vi "ROI entry-Check Z range and adjust.vi"(10 "ROI File data":dbl[][](array[numeric]), 11 "Old ROI file path":path) -> (2 "Adjusted ROI Data":dbl[][](array[numeric]), 3 "Latest AOL Z values":dbl[](array[numeric]))   [LabVIEW 2017]
uses:
  Typedefs/fgv_actions.ctl
panel:
  out "error out":errorcluster
  in  "error in (no error)":errorcluster
  in  "Loaded ROI Z Stop Values":dbl[](array[numeric])
  out "ROI Z stop (coerced)":dbl[](array[numeric])
  out "Z Stop Array":dbl[](array[numeric])
  out "Z Stop Code":u8[](array[numeric])
  out "Z start code":u8[](array[numeric])
  out "Z Start Array":dbl[](array[numeric])
  out "ROI Z start (coerced)":dbl[](array[numeric])
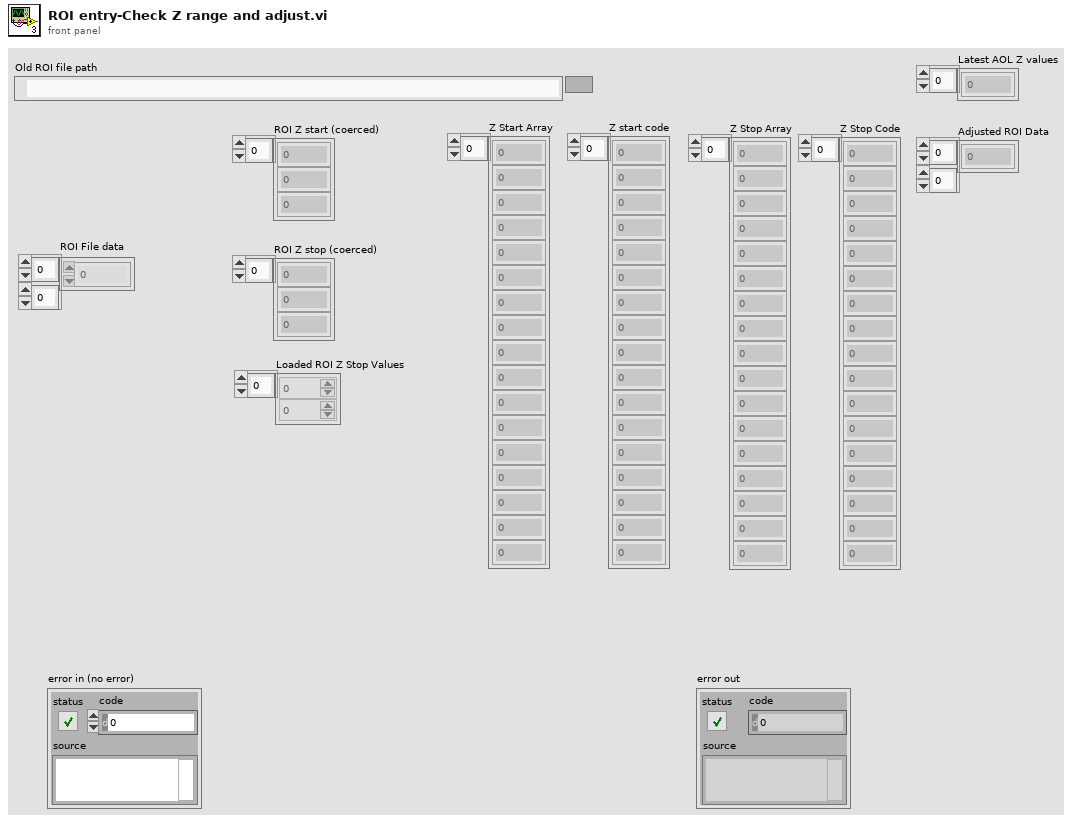
[diagram p1: front panel]
types:
  T1 = typedef "fgv_actions.ctl" = enum16{"Get", "Set"}
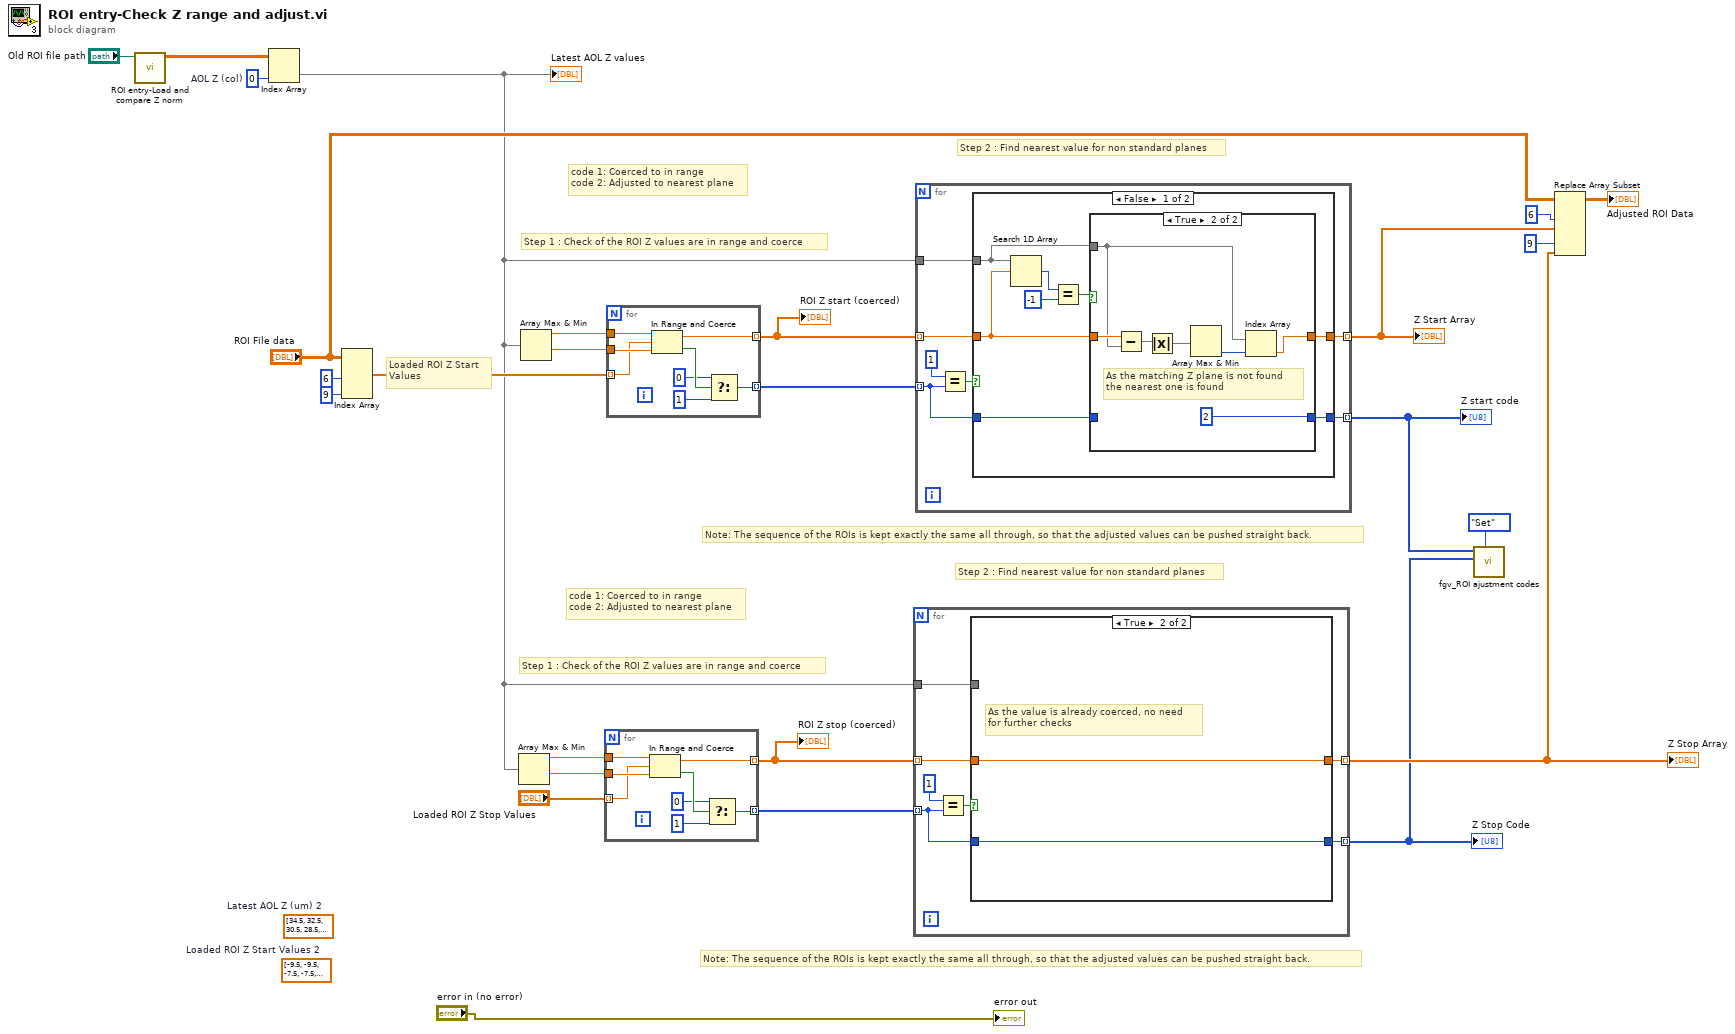
[diagram p0: block diagram]
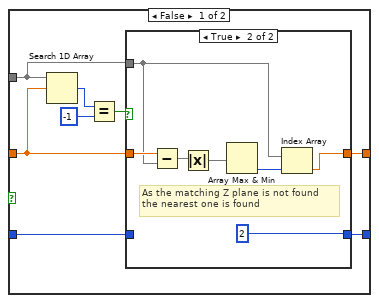
[diagram p2: hidden frame]
diagram:
  w6 = 0  # AOL Z (col)
  (unwired) dbl[] [-9.5, -9.5, -7.5, -7.5, -7.5, -7.5, -7.5, -7.5, -7.5, -7.5, -7.5, -7.5, -7.5, -7.5, -5.5, -3.5, -5.5, -5.5, -5.5, -5.5, -5.5, -5.5, -5.5, -3.5, -1.5, -1.5, -1.5, -1.5, -1.5, -1.5, -1.5, -1.5, -1.5, -3.5, -5.5, -7.5, -7.5, -7.5, -5.5, -5.5, -5.5, -5.5, -5.5, -5.5, -5.5, -3.5, -3.5, -3.5, -3.5, -1.5, -1.5, -1.5, -3.5, -7.5, -9.5, -15.5, -25.5, -31.5, -27.5, -17.5, -9.5, -5.5, -3.5, -3.5, -1.5, -1.5, -3.5, -5.5, -7.5, -9.5, -11.5, -9.5, -9.5, -5.5, -3.5, -3.5, -5.5, -5.5, -5.5, -3.5, -5.5, -5.5, -7.5, -9.5, -11.5, -9.5, -9.5, -7.5, -1.5, -1.5, -5.5, -7.5, -5.5, -3.5, -5.5, -5.5, -7.5, -7.5, -7.5, -9.5, -7.5, -5.5, -3.5, -3.5, -3.5, -7.5, -9.5]  # Loaded ROI Z Start Values 2
  (unwired) dbl[] [34.5, 32.5, 30.5, 28.5, 26.5, 24.5, 22.5, 20.5, 18.5, 16.5, 14.5, 12.5, 10.5, 8.5, 6.5, 4.5, 2.5, 0.5, -1.5, -3.5, -5.5, -7.5, -9.5, -11.5, -13.5, -15.5, -17.5, -19.5, -21.5, -23.5, -25.5, -27.5, -29.5, -31.5, -33.5, -35.5]  # Latest AOL Z (um) 2
  # "Loaded ROI Z Start \nValues"
  # "code 1: Coerced to in range\ncode 2: Adjusted to nearest plane"
  # "Note: The sequence of the ROIs is kept exactly the same all through, so that the adjusted values can be pushed straight back."
  # "Step 2 : Find nearest value for non standard planes"
  # "Step 1 : Check of the ROI Z values are in range and coerce"
  # "code 1: Coerced to in range\ncode 2: Adjusted to nearest plane"
  # "Note: The sequence of the ROIs is kept exactly the same all through, so that the adjusted values can be pushed straight back."
  # "Step 2 : Find nearest value for non standard planes"
  # "Step 1 : Check of the ROI Z values are in range and coerce"
  n1 = call "ROI entry-Load and compare Z norm.vi"("Old ROI file path"="Old ROI file path") -> ("Latest Zplane_Pockels_Values file data (header removed)"=w7:dbl[][])  [unwired: 4 in, 6 out]
  n2 = Index Array(array=w7, index (col)=w6) -> (element=w4:dbl[])  [unwired: 1 in]
  "Latest AOL Z values" <- w4
  n3 = Index Array(array="ROI File data", index (col) #1=6 ("disabled index (col)"), index (col) #2=9 ("index (col)")) -> (element #1=w14:dbl[])  [unwired: 2 in, 1 out]
  n4 = Array Max & Min(array=w4) -> (max value=w20:dbl, min value=w21:dbl)  [unwired: 2 out]
  n5 = Array Max & Min(array=w4) -> (max value=w25:dbl, min value=w24:dbl)  [unwired: 2 out]
  n6 = for {
    tunnel: "Loaded ROI Z Stop Values" -> [w32] mode=indexing
    tunnel: w20 -> [w34]
    tunnel: w21 -> [w33]
    tunnel: [w31] -> w19 mode=indexing
    tunnel: [w27] -> w22 mode=indexing
    n7 = In Range and Coerce(upper limit=w34, x=w32, lower limit=w33) -> (coerced(x)=w31:dbl, In Range?=w30:bool)
    n8 = Select(t=u8 0, s=w30, f=u8 1 ("t")) -> (s? t:f=w27:u8)
  }
  "ROI Z stop (coerced)" <- w19
  n9 = for {
    tunnel: w14 -> [w40] mode=indexing
    tunnel: w25 -> [w42]
    tunnel: w24 -> [w41]
    tunnel: [w39] -> w26 mode=indexing
    tunnel: [w35] -> w23 mode=indexing
    n10 = In Range and Coerce(upper limit=w42, x=w40, lower limit=w41) -> (coerced(x)=w39:dbl, In Range?=w38:bool)
    n11 = Select(t=u8 0, s=w38, f=u8 1 ("t")) -> (s? t:f=w35:u8)
  }
  "ROI Z start (coerced)" <- w26
  n12 = for {
    tunnel: w19 -> [w48] mode=indexing
    tunnel: w4 -> [w49]
    tunnel: [w47] -> w9 mode=indexing
    tunnel: w22 -> [w44] mode=indexing
    tunnel: [w43] -> w1 mode=indexing
    n13 = Equal?(x=u8 1 ("y"), y=w44) -> (x = y?=w46:bool)
    n14 = case shown="True" w46 {
      tunnel: w49 -> [w54 _]
      tunnel: w48 -> [w53 w68]
      tunnel: [w52 w68] -> w47
      tunnel: w44 -> [w51 w67]
      tunnel: [w50 w67] -> w43
      frame False {
        n15 = Search 1D Array(1D array=w54, element=w53) -> (index of element=w57:i32)  [unwired: 1 in]
        n16 = Equal?(x=w57, y=-1) -> (x = y?=w55:bool)
        n17 = case shown="True" w55 {
          tunnel: w54 -> [_ w65]
          tunnel: w53 -> [w59 w66]
          tunnel: [w59 w63] -> w52
          tunnel: w51 -> [w58 _]
          tunnel: [w58 u8 2] -> w50
          frame False {
            # "Matching Z plane is found in the\n AOL Z array, no adjustement needed"
          }
          frame True {
            # "As the matching Z plane is not found\nthe nearest one is found"
            n18 = Subtract(x=w66, y=w65) -> (x-y=w62:dbl[])
            n19 = Absolute Value(x=w62) -> (abs(x)=w61:dbl[])
            n20 = Array Max & Min(array=w61) -> (min index (indices)=w64:i32)  [unwired: 3 out]
            n21 = Index Array(array=w65, index=w64) -> (element=w63:dbl)
          }
        }
      }
      frame True {
        # "As the value is already coerced, no need \nfor further checks"
      }
    }
  }
  "Z Stop Array" <- w9
  "Z Stop Code" <- w1
  n22 = for {
    tunnel: w26 -> [w74] mode=indexing
    tunnel: w4 -> [w75]
    tunnel: [w73] -> w10 mode=indexing
    tunnel: w23 -> [w70] mode=indexing
    tunnel: [w69] -> w2 mode=indexing
    n23 = Equal?(x=u8 1 ("y"), y=w70) -> (x = y?=w72:bool)
    n24 = case shown="False" w72 {
      tunnel: w75 -> [w80 _]
      tunnel: w74 -> [w79 w94]
      tunnel: [w78 w94] -> w73
      tunnel: w70 -> [w77 w93]
      tunnel: [w76 w93] -> w69
      frame False {
        n25 = Search 1D Array(1D array=w80, element=w79) -> (index of element=w83:i32)  [unwired: 1 in]
        n26 = Equal?(x=w83, y=-1) -> (x = y?=w81:bool)
        n27 = case shown="True" w81 {
          tunnel: w80 -> [_ w91]
          tunnel: w79 -> [w85 w92]
          tunnel: [w85 w89] -> w78
          tunnel: w77 -> [w84 _]
          tunnel: [w84 u8 2] -> w76
          frame False {
            # "Matching Z plane is found in the\n AOL Z array, no adjustement needed"
          }
          frame True {
            # "As the matching Z plane is not found\nthe nearest one is found"
            n28 = Subtract(x=w92, y=w91) -> (x-y=w88:dbl[])
            n29 = Absolute Value(x=w88) -> (abs(x)=w87:dbl[])
            n30 = Array Max & Min(array=w87) -> (min index (indices)=w90:i32)  [unwired: 3 out]
            n31 = Index Array(array=w91, index=w90) -> (element=w89:dbl)
          }
        }
      }
      frame True {
        # "As the value is already coerced, no need \nfor further checks"
      }
    }
  }
  "Z Start Array" <- w10
  "Z start code" <- w2
  n32 = call "fgv_ROI ajustment codes.vi"("FGV Actions"=fgv_actions."Set", "Z stop codes IN"=w1, "Z start codes IN"=w2) -> ()  [unwired: 6 in, 3 out]
  n33 = Replace Array Subset(array="ROI File data", new element #1=w10, index (col) #1=6 ("disabled index (col)"), new element #2=w9, index (col) #2=9 ("index (col)")) -> (→"Adjusted ROI Data":dbl[][])  [unwired: 2 in]
  "error out" <- "error in (no error)"
